vi "TCSLINK_parserawstring.vi"(5 "Raw String":string) -> (2 "Array":string[](array[string]))   [LabVIEW 2015]
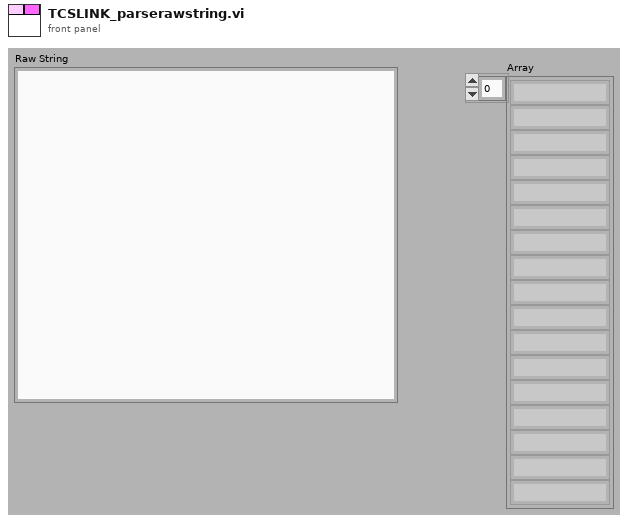
[diagram p1: front panel]
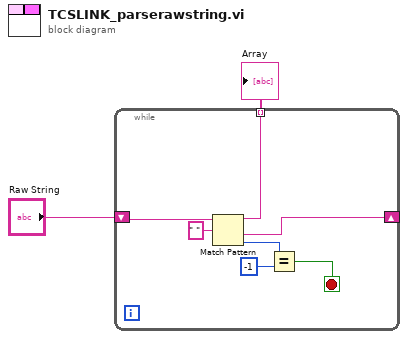
[diagram p0: block diagram]
diagram:
  n1 = while {
    shift-right: [w7] -> _
    shift-left: "Raw String" -> [w9]
    tunnel: [w6] -> w2 mode=indexing
    stop <- w5 stop-if-true
    n2 = Match Pattern(string=w9, regular expression=" ") -> (before substring=w6:string, after substring=w7:string, offset past match=w3:i32)  [unwired: 1 in, 1 out]
    n3 = Equal?(x=w3, y=-1) -> (x = y?=w5:bool)
  }
  "Array" <- w2
